vi "get map range.vi"(8 "error in (no error)":errorcluster, 11 "data array":string[](array[string])) -> (0 "error out":errorcluster, 2 "<JSON>":string[](array[string]) caption="<JSON>Items", 3 "Item Names":string[](array[string]))   [LabVIEW 2019]
uses:
  <vilib>/JDP Science/JSONtext/String Subset.vi
  <vilib>/JDP Science/JSONtext/support/Strip Quotes and Unescape.vi
  <vilib>/JDP Science/JSONtext/support/Unescape JSON string.vi
  <vilib>/JDP Science/JSONtext/Parsing/Parse Full Path or Item Name.vi
  <vilib>/JDP Science/JSONtext/Offset/Find Item Locations by Path.vi
  <vilib>/JDP Science/JSONtext/JSONtext.lvlib
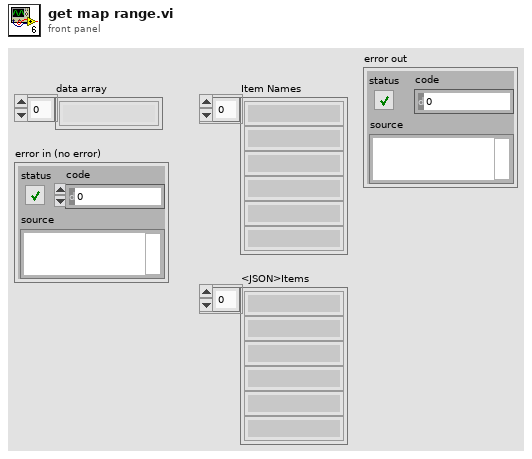
[diagram p1: front panel]
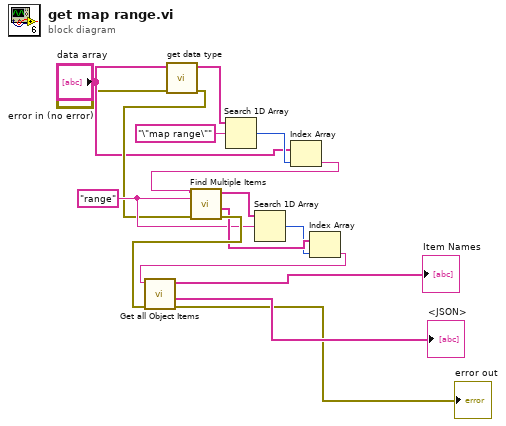
[diagram p0: block diagram]
diagram:
  w11 = "range" ("$Path or Item Name")
  n1 = call "get data type.vi"("error in (no error)"="error in (no error)", "data array"="data array") -> ("error out"=w8:errorcluster, "data type"=w3:string[])  [unwired: 8 in]
  n2 = Search 1D Array(1D array=w3, element="\"map range\"") -> (index of element=w6:i32)  [unwired: 1 in]
  n3 = Index Array(array="data array", index=w6) -> (element=w7:string)
  n4 = call <vilib>:"Find Multiple Items.vi"("$Path or Item Name"=w11, "error in (no error)"=w8, "JSON"=w7) -> ("error out"=w14:errorcluster, "<JSON>"=w12:string[], "Item Names"=w10:string[])  [unwired: 5 in, 1 out]
  n5 = Search 1D Array(1D array=w10, element=w11) -> (index of element=w9:i32)  [unwired: 1 in]
  n6 = Index Array(array=w12, index=w9) -> (element=w13:string)
  n7 = call <vilib>:"Get all Object Items.vi"("error in (no error)"=w14, "JSON"=w13) -> ("error out"=→"error out":errorcluster, "<JSON>"=→"<JSON>":string[], "Item Names"=→"Item Names":string[])  [unwired: 6 in, 1 out]
